vi "DevTests_ExeTTF.vi"() -> ()   [LabVIEW 2024]
uses:
  SDL3/Error/GetError-UiThread.vi
  <vilib>/Utility/error.llb/Error Cluster From Error Code.vi
  SDL3/Init/Init.lvlib
  SDL3/TTF/TTF.lvlib
panel:
  out "error out":errorcluster
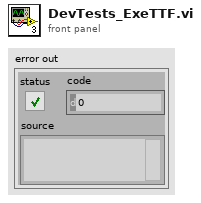
[diagram p1: front panel]
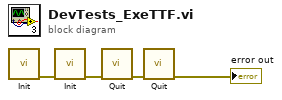
[diagram p0: block diagram]
diagram:
  n1 = call "Init.vi"() -> ("error out"=w4:errorcluster)  [unwired: 11 in]
  n2 = call "Init.vi"("No Error"=w4) -> ("error out"=w3:errorcluster)  [unwired: 10 in]
  n3 = call "Quit.vi"("No Error"=w3) -> ("error out"=w2:errorcluster)  [unwired: 10 in]
  n4 = call "Quit.vi"("No Error"=w2) -> ("error out"=→"error out":errorcluster)  [unwired: 10 in]
